vi "Initialization VI.vi"(8 "error in (no error)":errorcluster, 10 "Custom XML":string, 11 "Device Item Ref in":T1 format="%.0x") -> (0 "error out":errorcluster, 3 "Device Item Ref out":T1 format="%.0x")   [LabVIEW 2014, in "PXIe 4113 System Explorer.lvlib"]
uses:
  PXIe 4113 System Explorer.lvlib
  <vilib>/NI Veristand/Custom Device API/Custom Device Item Ref.ctl
  <vilib>/NI Veristand/Custom Device API/Custom Device Channel.ctl
  <vilib>/NI Veristand/Custom Device API/Custom Device Channel Type.ctl
  <vilib>/NI Veristand/Custom Device API/Custom Device API.lvlib
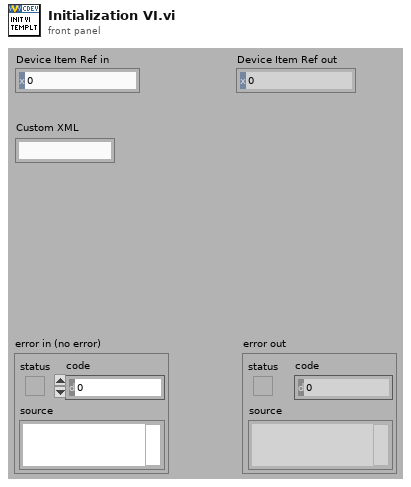
[diagram p1: front panel]
types:
  T1 = typedef "Custom Device API.lvlib/Custom Device Item Ref.ctl" = u64
  T2 = typedef "Custom Device API.lvlib/Custom Device Channel.ctl" = cluster{"Type":T3, "Units":string, "Default Value":dbl, "Faultable":bool, "Scalable":bool}
  T3 = typedef "Custom Device API.lvlib/Custom Device Channel Type.ctl" = enum16{"Input", "Output"}
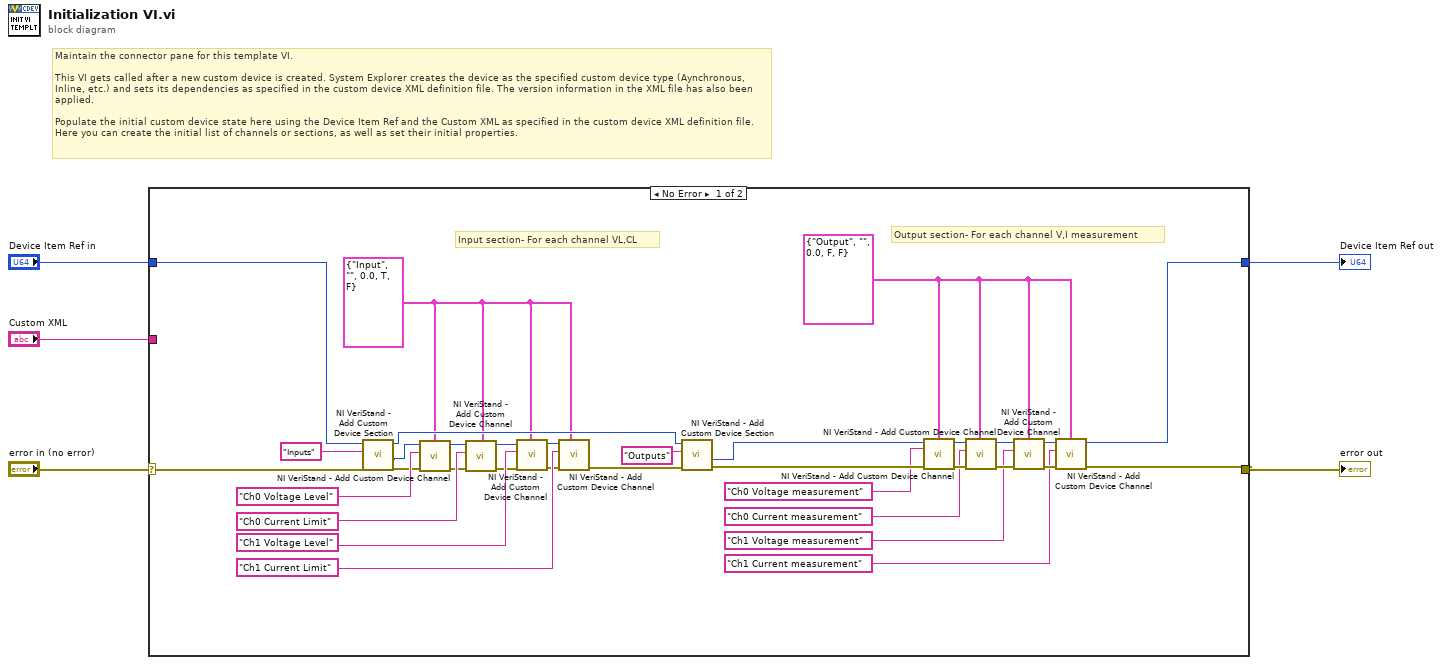
[diagram p0: block diagram]
diagram:
  # "Maintain the connector pane for this template VI.\n\nThis VI gets called after a new custom device is created. System Explorer creates the device as the specified custom device type (Aynchronous, Inline, etc.) and sets its dependencies as specified in the custom device XML definition file. The version information in the XML file has also been applied.\n\nPopulate the initial custom device state here using the Device Item Ref and the Custom XML as specified in the custom device XML definition file. Here you can create the initial list of channels or sections, as well as set their initial properties."
  n1 = case shown="No Error" "error in (no error)" {
    selector: "error in (no error)" -> [w8 w41]
    tunnel: [w7 w41] -> w5
    tunnel: [w6 w40] -> w3
    tunnel: "Device Item Ref in" -> [w9 w40]
    tunnel: "Custom XML" -> [_ _]
    frame No Error {
      w33 = T2 {"Type"=enum."Output", "Units"="", "Default Value"=0.0, "Faultable"=FALSE, "Scalable"=FALSE} ("Channel")
      w32 = T2 {"Type"=enum."Input", "Units"="", "Default Value"=0.0, "Faultable"=TRUE, "Scalable"=FALSE} ("Channel")
      # "Output section- For each channel V,I measurement"
      # "Input section- For each channel VL,CL"
      n2 = call <vilib>:"NI VeriStand - Add Custom Device Section.vi"("error in (no error)"=w8, "Section Name"="Inputs", "Parent Ref in"=w9) -> ("error out"=w11:errorcluster, "Section Ptr"=w37:T1, "Parent Ref out"=w38:T1)  [unwired: 5 in, 1 out]
      n3 = call <vilib>:"NI VeriStand - Add Custom Device Channel.vi"("error in (no error)"=w11, "Channel"=w32, "Channel Name"="Ch0 Voltage Level", "Parent Ref in"=w37) -> ("error out"=w12:errorcluster, "Parent Ref out"=w13:T1)  [unwired: 4 in, 2 out]
      n4 = call <vilib>:"NI VeriStand - Add Custom Device Channel.vi"("error in (no error)"=w12, "Channel"=w32, "Channel Name"="Ch0 Current Limit", "Parent Ref in"=w13) -> ("error out"=w17:errorcluster, "Parent Ref out"=w16:T1)  [unwired: 4 in, 2 out]
      n5 = call <vilib>:"NI VeriStand - Add Custom Device Channel.vi"("error in (no error)"=w17, "Channel"=w32, "Channel Name"="Ch1 Voltage Level", "Parent Ref in"=w16) -> ("error out"=w14:errorcluster, "Parent Ref out"=w15:T1)  [unwired: 4 in, 2 out]
      n6 = call <vilib>:"NI VeriStand - Add Custom Device Channel.vi"("error in (no error)"=w14, "Channel"=w32, "Channel Name"="Ch1 Current Limit", "Parent Ref in"=w15) -> ("error out"=w36:errorcluster)  [unwired: 4 in, 3 out]
      n7 = call <vilib>:"NI VeriStand - Add Custom Device Section.vi"("error in (no error)"=w36, "Section Name"="Outputs", "Parent Ref in"=w38) -> ("error out"=w31:errorcluster, "Section Ptr"=w39:T1)  [unwired: 5 in, 2 out]
      n8 = call <vilib>:"NI VeriStand - Add Custom Device Channel.vi"("error in (no error)"=w31, "Channel"=w33, "Channel Name"="Ch0 Voltage measurement", "Parent Ref in"=w39) -> ("error out"=w29:errorcluster, "Parent Ref out"=w30:T1)  [unwired: 4 in, 2 out]
      n9 = call <vilib>:"NI VeriStand - Add Custom Device Channel.vi"("error in (no error)"=w29, "Channel"=w33, "Channel Name"="Ch0 Current measurement", "Parent Ref in"=w30) -> ("error out"=w26:errorcluster, "Parent Ref out"=w25:T1)  [unwired: 4 in, 2 out]
      n10 = call <vilib>:"NI VeriStand - Add Custom Device Channel.vi"("error in (no error)"=w26, "Channel"=w33, "Channel Name"="Ch1 Voltage measurement", "Parent Ref in"=w25) -> ("error out"=w28:errorcluster, "Parent Ref out"=w27:T1)  [unwired: 4 in, 2 out]
      n11 = call <vilib>:"NI VeriStand - Add Custom Device Channel.vi"("error in (no error)"=w28, "Channel"=w33, "Channel Name"="Ch1 Current measurement", "Parent Ref in"=w27) -> ("error out"=w7:errorcluster, "Parent Ref out"=w6:T1)  [unwired: 4 in, 2 out]
    }
    frame Error {
    }
  }
  "error out" <- w5
  "Device Item Ref out" <- w3
